vi "UE9 DO Port Update Loop.vi"() -> ()   [LabVIEW 2021]
panel:
  in  "Values":u16[](array[numeric])=[0, 65535, 0, 43690, 0, 65535, 0, 43690]
  out "Iteration#":i32
  in  "Interval [ms]":u32=500
  out "Error Message":string
  out "error out":errorcluster
  # "Outputs an array of 16-bit values to FIO & EIO.  Each iteration the digital outputs are\nupdated with a value from the array."
  # "The first 16-bits of DO will be set to b0000000000000000, then 500ms\nlater will be set to b1111111111111111, then 500ms later will be set\nto b0000000000000000, then 500ms later will be set to b1010101010101010,\n... and so on."
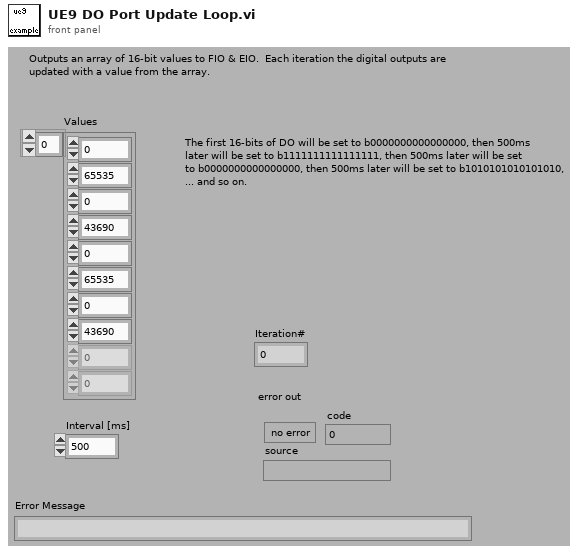
[diagram p1: front panel]
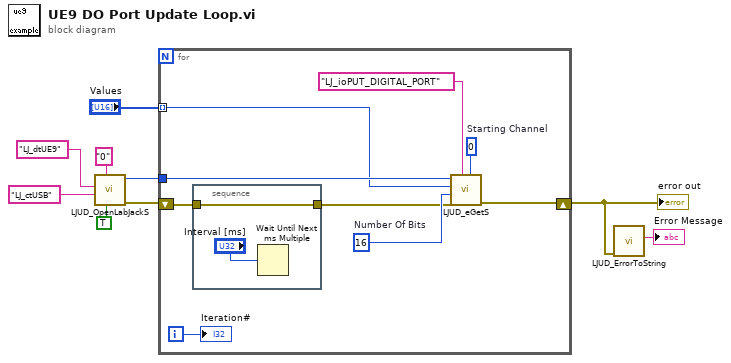
[diagram p0: block diagram]
diagram:
  n1 = call "LJUD_OpenLabJackS.vi"("FirstFound"=TRUE, "Address"="0", "ConnectionType"="LJ_ctUSB", "DeviceType"="LJ_dtUE9") -> ("error out"=w3:errorcluster, "Handle"=w2:i32)  [unwired: 5 in, 1 out]
  n2 = for {
    shift-right: [w16] -> w4
    shift-left: w3 -> [w11]
    tunnel: w2 -> [w15]
    tunnel: "Values" -> [w14] mode=indexing
    i -> [w17]
    w12 = 0  # Starting Channel
    w13 = 16  # Number Of Bits
    n3 = stacked-sequence {
      tunnel: w11 -> [w19]
      tunnel: [w19] -> w10
      frame #0 {
        n4 = Wait Until Next ms Multiple(millisecond multiple="Interval [ms]") -> ()  [unwired: 1 out]
      }
    }
    n5 = call "LJUD_eGetS.vi"("Channel"=w12, "IOType"="LJ_ioPUT_DIGITAL_PORT", "error in"=w10, "x1"=w13, "Value Write"=w14, "Handle In"=w15) -> ("error out"=w16:errorcluster)  [unwired: 3 in, 2 out]
    "Iteration#" <- w17
  }
  "error out" <- w4
  n6 = call "LJUD_ErrorToString.vi"("error in"=w4) -> ("String"=→"Error Message":string)  [unwired: 10 in]
